vi "PicoScope6000Open.vi"(7 "Mode":u16(ring) items=["Dialog On Error", "no dialog - CloseUnit and Stop", "no dialog - Continue", "no dialog - Stop"], 8 "error in (no error)":errorcluster, 9 "Serial Number":string, 10 "Use Serial Number":bool) -> (0 "error out":errorcluster, 1 "Max Adc value":i16, 3 "handle":i16, 4 "Device Info":T1, 6 "Pico 6000 Units":string)   [LabVIEW 2009]
doc: "This VI opens a PicoScope 6000 and returns a handle to the device."
uses:
  ps6000.dll
panel:
  out "serialLth":i16
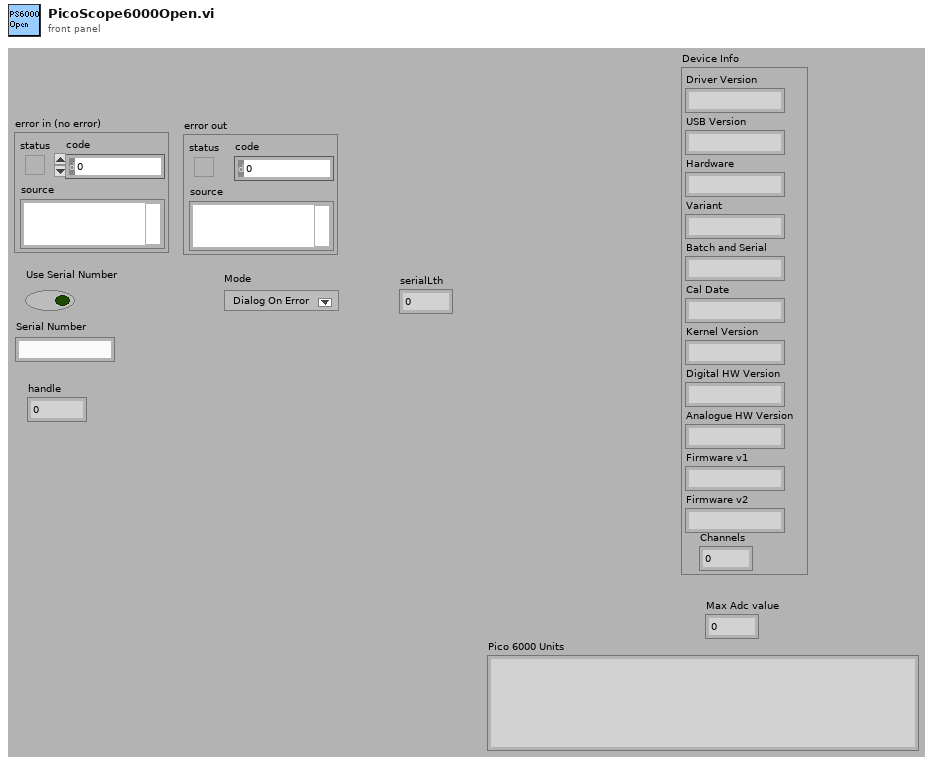
[diagram p1: front panel]
types:
  T1 = cluster{"Driver Version":string, "USB Version":string, "Hardware":string, "Variant":string, "Batch and Serial":string, "Cal Date":string, "Kernel Version":string, "Digital HW Version":string, "Analogue HW Version":string, "Firmware v1":string, "Firmware v2":string, "Channels":i16}
  T2 = cluster{"status":bool, "code":u32, "source":string}
  T3 = cluster{"Driver Version":string, "USB Version":string, "Hardware":string, "Variant":string, "Batch and Serial":string, "Cal Date":string, "Kernel Version":string, "Digital HW Version":string, "Analogue HW Version":string, "Firmware v1":string, "Firmware v2":string}
  T4 = cluster{"Driver Version":string, "USB Version":string, "Hardware":string, "Variant":string, "Batch and Serial":string, "Cal Date":string, "Kernel Version":string, "Digital HW Version":string, "Analogue HW Version":string, "Firmware v1":string, "Firmware v2":string, i16}
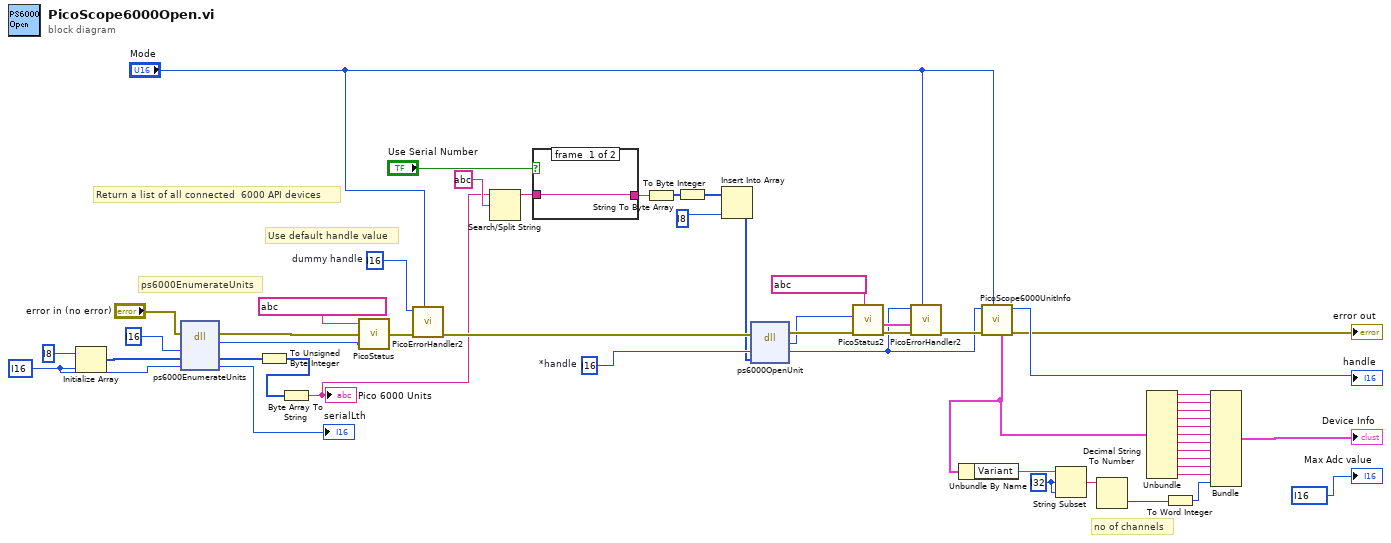
[diagram p0: block diagram]
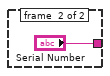
[diagram p2: hidden frame]
diagram:
  w18 = i16 ?  # dummy handle
  w22 = i16 ? ("dimension size")
  w34 = i32 ? ("offset (0)")
  w16 = i16 ?  # *handle
  # "Use default handle value"
  # "Return a list of all connected  6000 API devices"
  # "ps6000EnumerateUnits"
  # "no of channels"
  n1 = Initialize Array(i8 ? ("U8"), w22) -> (w24:i8[])
  n2 = dll-call lib="ps6000.dll" fn="ps6000EnumerateUnits"(error in="error in (no error)", "count"=i16 ?, "serials"=w24, "serialLth"=w22) -> (error out=w29:errorcluster, "PICO_STATUS"=w28:u32, "serials"=w20:i8[], "serialLth"=→"serialLth":i16)  [unwired: 3 in, 1 out]
  n3 = To Unsigned Byte Integer(number=w20) -> (unsigned 8bit integer=w21:u8[])
  n4 = Byte Array To String(unsigned byte array=w21) -> (string=w3:string)
  "Pico 6000 Units" <- w3
  n5 = call "PicoStatus.vi"("PICO STATUS"=w28, "error in"=w29, "source"=string ?) -> ("error out"=w19:errorcluster)
  n6 = call "PicoErrorHandler2.vi"("Mode"="Mode", "error in (no error)"=w19, "handle In"=w18) -> ("error out"=w17:errorcluster)  [unwired: 8 in]
  n7 = Search/Split String(string=w3, search string/char (-)=string ?) -> (substring before match=w11:string)  [unwired: 1 in, 2 out]
  n8 = case shown="True" "Use Serial Number" {
    tunnel: w11 -> [w54 _]
    tunnel: [w54 "Serial Number"] -> w7
    frame #0 {
    }
    frame #1 {
    }
  }
  n9 = String To Byte Array(string=w7) -> (unsigned byte array=w9:u8[])
  n10 = To Byte Integer(number=w9) -> (8bit integer=w10:i8[])
  n11 = Insert Into Array(array=w10, new element=i8 ? ("new element/subarray")) -> (w6:i8[])  [unwired: 1 in]
  n12 = dll-call lib="PS6000.dll" fn="ps6000OpenUnit" ("ps3000.dll:_ps3000_open_unit@0")(error in=w17, "handle"=w16, "serial"=w6) -> (error out=w15:errorcluster, "PICO_STATUS"=w14:u32, "handle"=w13:i16)  [unwired: 3 in, 1 out]
  n13 = call "PicoStatus2.vi"("PICO source"=string ? ("source"), "Error in"=w15, "PICO STATUS"=w14) -> ("error out"=w39:errorcluster, "PICO_STATUS out"=w38:T2)  [unwired: 5 in]
  n14 = call "PicoErrorHandler2.vi"("Mode"="Mode", "error in (no error)"=w39, "PICO_STATUS in"=w38, "handle In"=w13) -> ("error out"=w37:errorcluster)  [unwired: 7 in]
  n15 = call "PicoScope6000UnitInfo.vi"("Mode"="Mode", "error in (no error)"=w37, "handle in"=w13) -> ("error out"=→"error out":errorcluster, "handle out"=→"handle":i16, "Unit Info"=w2:T3)  [unwired: 6 in]
  n16 = Unbundle By Name(w2) -> ("Variant"=w31:string)
  n17 = String Subset(string=w31, offset (0)=w34, length (rest)=w34) -> (substring=w33:string)
  n18 = Decimal String To Number(string=w33) -> (number=w32:i32)  [unwired: 2 in, 1 out]
  n19 = Unbundle(w2) -> ("Driver Version"=w51:string, "USB Version"=w50:string, "Hardware"=w49:string, "Variant"=w48:string, "Batch and Serial"=w47:string, "Cal Date"=w46:string, "Kernel Version"=w45:string, "Digital HW Version"=w44:string, "Analogue HW Version"=w43:string, "Firmware v1"=w42:string, "Firmware v2"=w41:string)
  n20 = To Word Integer(number=w32) -> (16bit integer=w30:i16)
  n21 = Bundle("Driver Version"=w51, "USB Version"=w50, "Hardware"=w49, "Variant"=w48, "Batch and Serial"=w47, "Cal Date"=w46, "Kernel Version"=w45, "Digital HW Version"=w44, "Analogue HW Version"=w43, "Firmware v1"=w42, "Firmware v2"=w41, w30) -> (→"Device Info":T4)  [unwired: 1 in]
  "Max Adc value" <- i16 ? ("Max Adc value")
